vi "SysLog Code 2 Message with Parameters.vi"(6 "cRIO":bool, 11 "Array-Typ (2D Dbl) (Eingang)":string[][](array[string])) -> (3 "Array-Typ (2D Dbl) (Ausgang)":string[][](array[string]))   [LabVIEW 2020, in "SysLog.lvlib"]
uses:
  SysLog.lvlib
  Sprachverwaltung/FGV Aktion Tabelle zerlegen.ctl
  Seiten/System Einstellungen V2/Aktioen FGV System Konstanten.ctl
  Sprachverwaltung/Sprachverwaltung.lvlib
  Seiten/System Einstellungen V2/System Einstellungen V2.lvlib
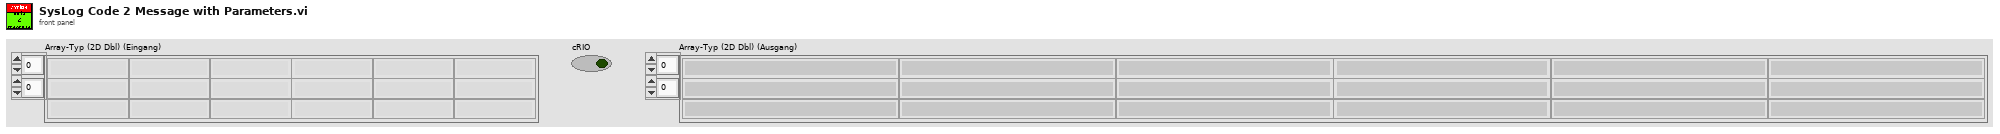
[diagram p1: front panel]
types:
  T1 = typedef "System Einstellungen V2.lvlib/Aktioen FGV System Konstanten.ctl" = enum16{"lesen", "laden", "speichern", "Sprache"}
  T2 = typedef "Sprachverwaltung.lvlib/FGV Aktion Tabelle zerlegen.ctl" = enum16{"laden", "vereinzeln", "speichern"}
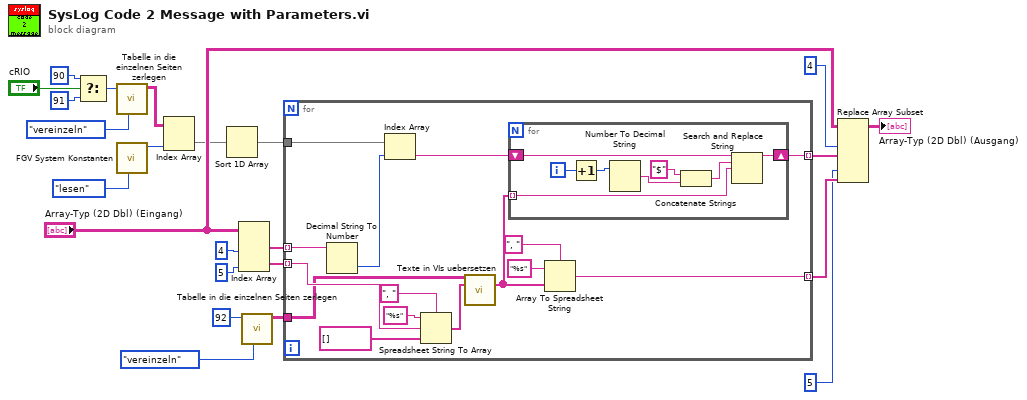
[diagram p0: block diagram]
diagram:
  n1 = Select(t=90, s="cRIO", f=91 ("Index (Seite)")) -> (s? t:f=w3:i32)
  n2 = call "Tabelle in die einzelnen Seiten zerlegen.vi"("Aktion"=FGV_Aktion_Tabelle_zerlegen."vereinzeln", "Index (Seite)"=w3) -> ("Sprachliste"=w12:string[][])  [unwired: 7 in, 2 out]
  n3 = call "FGV System Konstanten.vi"("Aktionen"=Aktioen_FGV_System_Konstanten."lesen") -> ("Sprachindex"=w5:u16)  [unwired: 6 in, 4 out]
  n4 = Index Array(array=w12, index (col)=w5) -> (element=w11:string[])  [unwired: 1 in]
  n5 = Sort 1D Array(array=w11) -> (sorted array=w10:string[])
  n6 = Index Array(array="Array-Typ (2D Dbl) (Eingang)", index (col) #1=4 ("Deaktivierter Index (Spalte)"), index (col) #2=5 ("Index (Spalte)")) -> (element #1=w18:string[], element #2=w8:string[])  [unwired: 2 in]
  n7 = call "Tabelle in die einzelnen Seiten zerlegen.vi"("Aktion"=FGV_Aktion_Tabelle_zerlegen."vereinzeln", "Index (Seite)"=92) -> ("Sprachliste"=w7:string[][])  [unwired: 7 in, 2 out]
  n8 = for {
    tunnel: w18 -> [w38] mode=indexing
    tunnel: [w28] -> w16 mode=indexing
    tunnel: w10 -> [w37]
    tunnel: w8 -> [w35] mode=indexing
    tunnel: w7 -> [w31]
    tunnel: [w24] -> w6 mode=indexing
    n9 = Decimal String To Number(string=w38) -> (number=w36:i32)  [unwired: 2 in, 1 out]
    n10 = Index Array(array=w37, index=w36) -> (element=w29:string)
    n11 = Spreadsheet String To Array(delimiter (Tab)=", " ("Trennzeichen (Tabulator)"), format string="%s" ("Format-String"), spreadsheet string=w35, array type (2D Dbl)=string[] []) -> (array=w30:string[])
    n12 = call "Texte in VIs uebersetzen.vi"("Sprachliste"=w31, "String-Array zum Übersetzen"=w30) -> ("String-Array zum Übersetzen"=w27:string[])  [unwired: 9 in, 4 out]
    n13 = for {
      tunnel: w27 -> [w46] mode=indexing
      shift-right: [w39] -> w28
      shift-left: w29 -> [w45]
      i -> [w42]
      n14 = Increment(x=w42) -> (x+1=w41:i32)
      n15 = Number To Decimal String(number=w41) -> (decimal integer string=w40:string)  [unwired: 1 in]
      n16 = Concatenate Strings("$" ("Such-String"), w40) -> (w43:string)
      n17 = Search and Replace String(input string=w45, search string=w43, replace string=w46) -> (result string=w39:string)  [unwired: 5 in, 3 out]
    }
    n18 = Array To Spreadsheet String(delimiter (Tab)=", " ("Trennzeichen (Tabulator)"), array=w27, 3:"%s" ("Format-String")) -> (spreadsheet string=w24:string)
  }
  n19 = Replace Array Subset(array="Array-Typ (2D Dbl) (Eingang)", new element #1=w16, index (col) #1=4 ("Deaktivierter Index (Spalte)"), new element #2=w6, index (col) #2=5 ("Index (Spalte)")) -> (→"Array-Typ (2D Dbl) (Ausgang)":string[][])  [unwired: 2 in]
